vi "Read limit_alarm_max.vi"(8 "error in (no error)":errorcluster caption="entrée d'erreur (pas d'erreur)", 11 "DAQmxTaskAICurrent en entrée":refnum<class "DAQmxTaskAICurrent.lvclass">) -> (0 "error out":errorcluster caption="sortie d'erreur", 2 "limit_alarm_max":dbl, 3 "DAQmxTaskAICurrent en sortie":refnum<class "DAQmxTaskAICurrent.lvclass">)   [LabVIEW 2015, in "DAQmxTaskAICurrent.lvclass"]
uses:
  DAQmxTaskAICurrent.lvclass
  DAQmxTaskAICurrent.lvclass/DAQmxTaskAICurrent.ctl
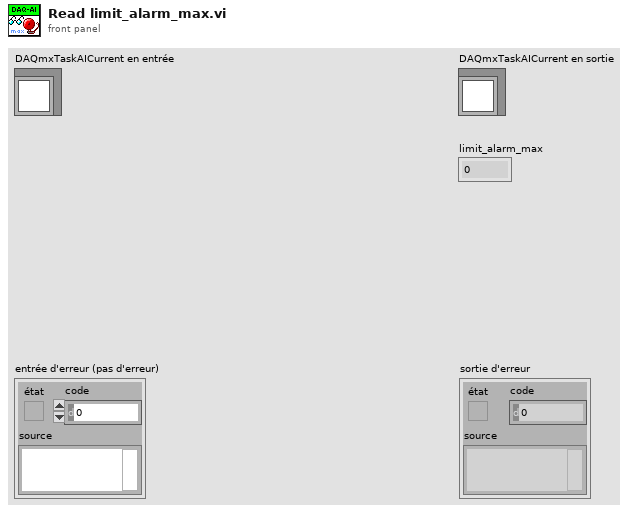
[diagram p1: front panel]
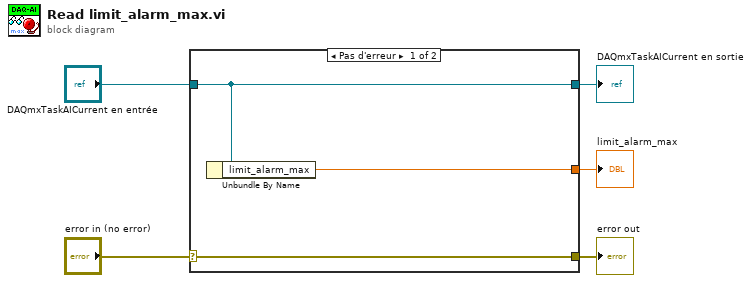
[diagram p0: block diagram]
diagram:
  n1 = case shown="Pas d'erreur" "error in (no error)" {
    selector: "error in (no error)" -> [w8 w9]
    tunnel: [w8 w9] -> w4
    tunnel: [w7 w10] -> w2
    tunnel: "DAQmxTaskAICurrent en entrée" -> [w7 w10]
    tunnel: [w6 _] -> w1
    frame No Error {
      n2 = Unbundle By Name(w7) -> ("limit_alarm_max"=w6:dbl)
    }
    frame Error {
    }
  }
  "error out" <- w4
  "DAQmxTaskAICurrent en sortie" <- w2
  "limit_alarm_max" <- w1
